vi "MessageBox.vi"(3 "error in (no error)":errorcluster, 4 "String":string) -> (0 "error out":errorcluster, 1 "This VI":refnum<vi>)   [LabVIEW 2015]
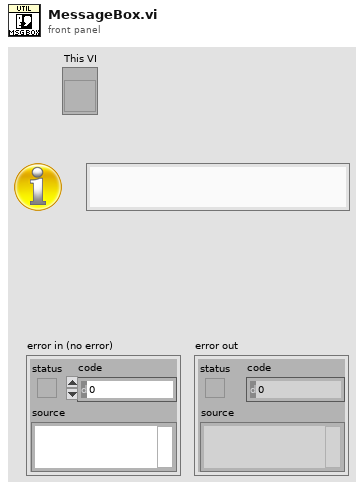
[diagram p1: front panel]
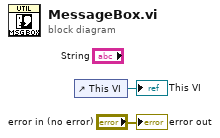
[diagram p0: block diagram]
diagram:
  n1 = control-ref of="This VI"() -> (→"This VI":refnum<vi>)
  "error out" <- "error in (no error)"
